vi "Clear Log Control.vi"(8 "エラー入力 (エラーなし)":errorcluster, 11 "Control“ü—Í":refnum<vi>) -> (0 "エラー出力":errorcluster)   [LabVIEW 2014]
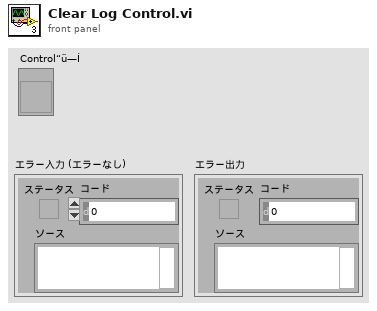
[diagram p1: front panel]
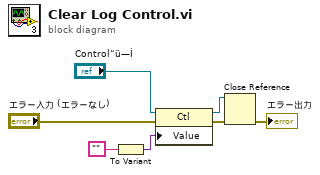
[diagram p0: block diagram]
diagram:
  n1 = To Variant(anything="") -> (Variant=w6:variant)
  n2 = property class="Ctl"(reference="Control“ü—Í", error in="エラー入力 (エラーなし)", "Value"=w6) -> (reference out=w5:refnum<vi>, error out=w4:errorcluster)
  n3 = Close Reference(reference=w5, error in (no error)=w4) -> (error out=→"エラー出力":errorcluster)
